vi "Pressure Cal UI.vi"() -> ()   [LabVIEW 2012]
panel:
  in  "f0":cluster{dbl, dbl}[](graph)
  in  "Q":cluster{dbl, dbl}[](graph)
  in  "P":cluster{dbl, dbl}[](graph)
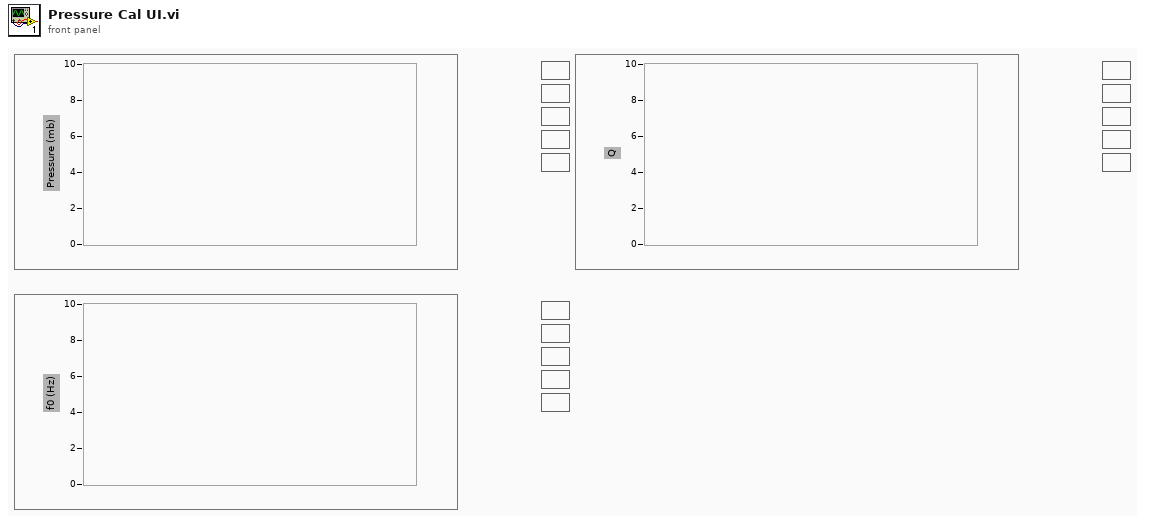
[diagram p1: front panel]
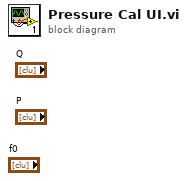
[diagram p0: block diagram]
diagram:
